vi "About.vi"() -> ()   [LabVIEW 2015, in "Application.lvclass"]
uses:
  Application.lvclass
panel:
  out "Author":string
  out "App_Info":string
  out "Logo":picture
  in  "Btn":bool
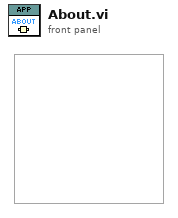
[diagram p1: front panel]
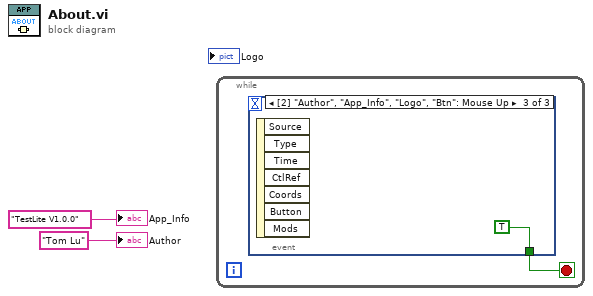
[diagram p0: block diagram]
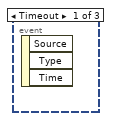
[diagram p2: hidden frame]
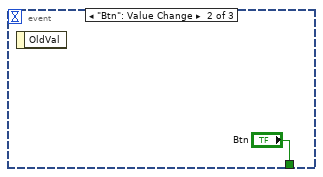
[diagram p3: hidden frame]
diagram:
  n1 = while {
    stop <- w3 stop-if-true
    n2 = event shown="[2] \"Author\", \"App_Info\", \"Logo\", \"Btn\": Mouse Up" {
      selector: _ -> [_ _ _]
      dyn-events: _ -> [_ _ _]
      timeout: _ -> [_ _ _]
      tunnel: [_ "Btn" TRUE] -> w3
      event Timeout {
        n3 = event-data() -> ()  [unwired: 1 in, 3 out]
      }
      event "Btn": Value Change {
        n4 = event-data() -> ()  [unwired: 1 in, 1 out]
      }
      event "Author", "App_Info", "Logo", "Btn": Mouse Up {
        n5 = event-data() -> ()  [unwired: 1 in, 7 out]
      }
    }
  }
  "App_Info" <- "TestLite V1.0.0"
  "Author" <- "Tom Lu" ("Author")
